vi "DataStorageSendDataEventRoutedMessage_Parse.vi"(8 "error in (no error)":errorcluster, 11 "Message":T10) -> (0 "error out":errorcluster, 1 "Body":T1, 2 "Header":T9, 3 "DataStorageSendDataEventRoutedMessage":T8)   [LabVIEW 2017]
uses:
  <vilib>/addons/InsightCM/MessageBus/Base/controls/Message.ctl
  <vilib>/addons/InsightCM/MessageBus/Base/controls/MessageHeader.ctl
  <vilib>/addons/InsightCM/MessageBus/Base/controls/KeyValuePair.ctl
  <vilib>/addons/InsightCM/MessageBus/MessageLibrary/DataStorage/controls/DataStorageSendDataEventRoutedMessage.ctl
  <vilib>/addons/InsightCM/MessageBus/MessageLibrary/DataStorage/controls/DataStorageSendDataEventRoutedMessageBody.ctl
  <vilib>/addons/InsightCM/MessageBus/Base/controls/DataEvent.ctl
  <vilib>/addons/InsightCM/MessageBus/Base/controls/DataSetMetadata.ctl
  <vilib>/addons/InsightCM/MessageBus/Base/controls/TrendPoint.ctl
  <vilib>/addons/InsightCM/MessageBus/Base/controls/TrendAlarmUpdate.ctl
  <vilib>/addons/InsightCM/MessageBus/Base/controls/TrendAlarmTransition.ctl
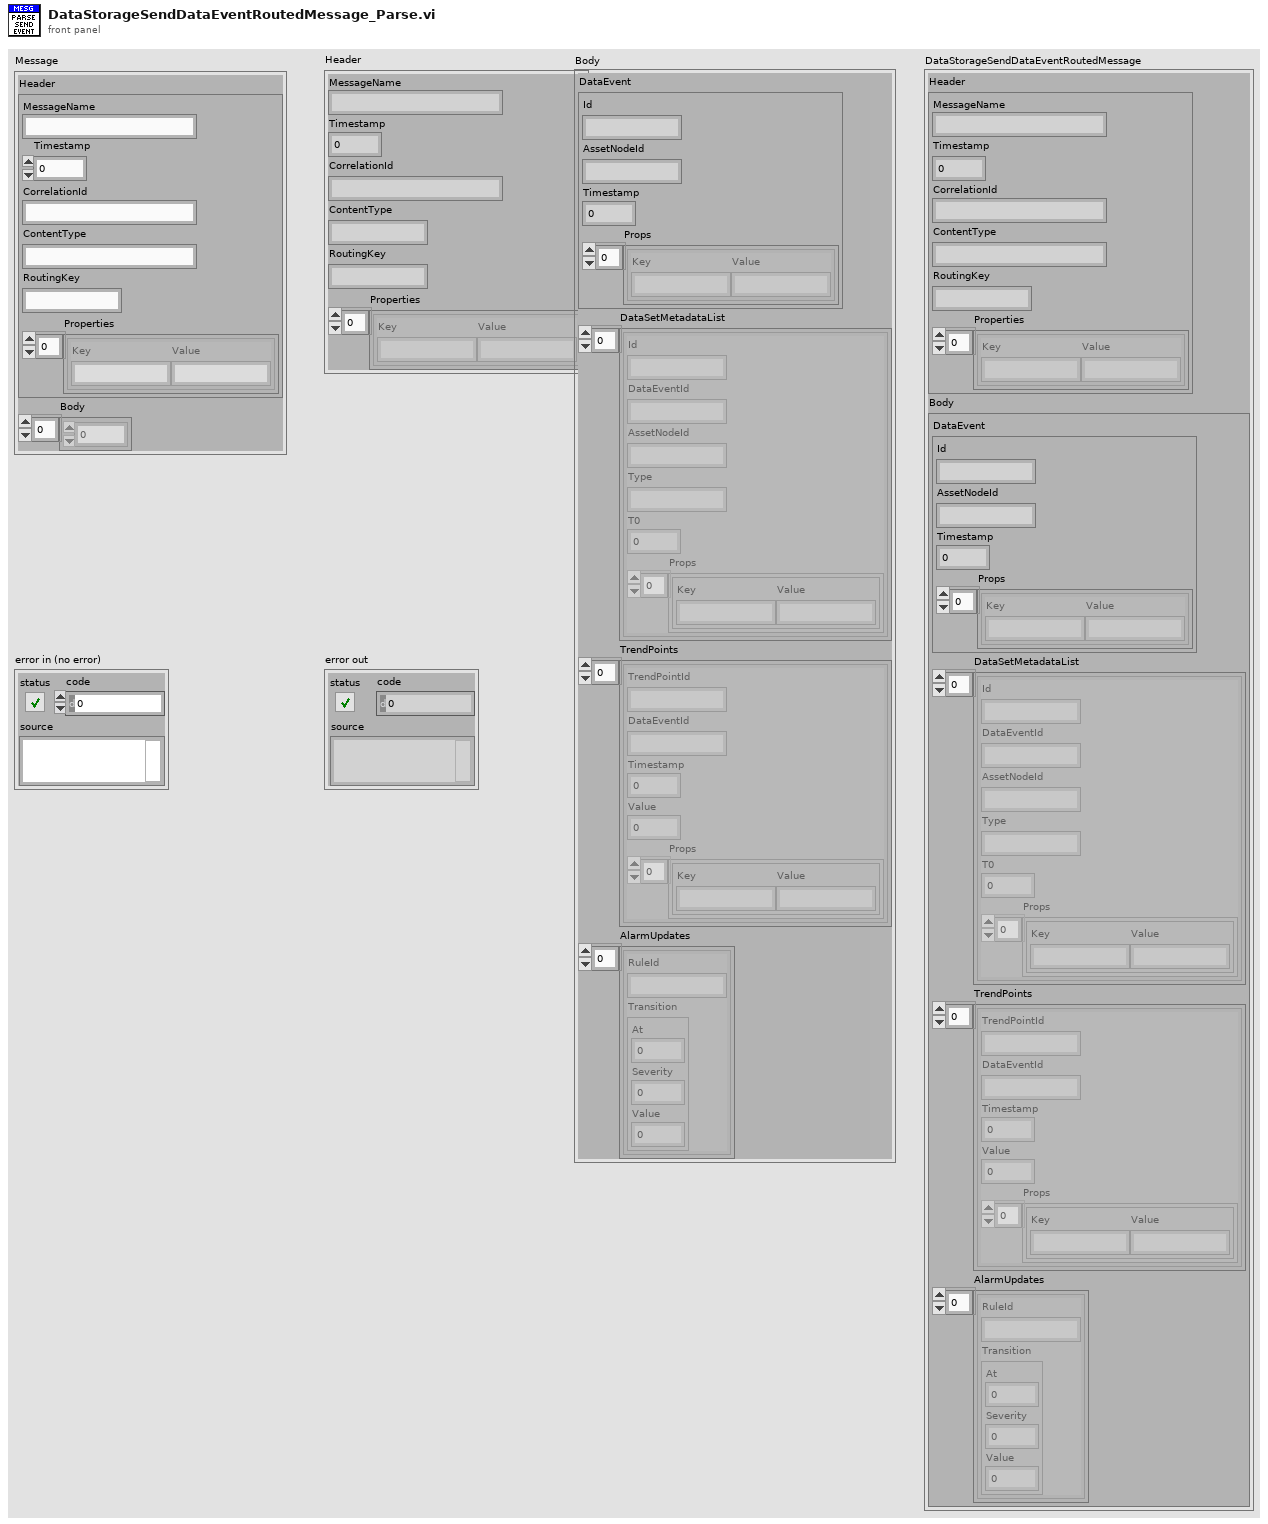
[diagram p1: front panel]
types:
  T1 = typedef "DataStorageSendDataEventRoutedMessageBody.ctl" = cluster{"DataEvent":T2, "DataSetMetadataList":T4[], "TrendPoints":T5[], "AlarmUpdates":T6[]}
  T2 = typedef "DataEvent.ctl" = cluster{"Id":string, "AssetNodeId":string, "Timestamp":i64, "Props":T3[]}
  T3 = typedef "KeyValuePair.ctl" = cluster{"Key":string, "Value":string}
  T4 = typedef "DataSetMetadata.ctl" = cluster{"Id":string, "DataEventId":string, "AssetNodeId":string, "Type":string, "T0":i64, "Props":T3[]}
  T5 = typedef "TrendPoint.ctl" = cluster{"TrendPointId":string, "DataEventId":string, "Timestamp":i64, "Value":dbl, "Props":T3[]}
  T6 = typedef "TrendAlarmUpdate.ctl" = cluster{"RuleId":string, "Transition":T7}
  T7 = typedef "TrendAlarmTransition.ctl" = cluster{"At":i64, "Severity":i32, "Value":dbl}
  T8 = typedef "DataStorageSendDataEventRoutedMessage.ctl" = cluster{"Header":T9, "Body":T1}
  T9 = typedef "MessageHeader.ctl" = cluster{"MessageName":string, "Timestamp":i64, "CorrelationId":string, "ContentType":string, "RoutingKey":string, "Properties":T3[]}
  T10 = typedef "Message.ctl" = cluster{"Header":T9, "Body":u8[]}
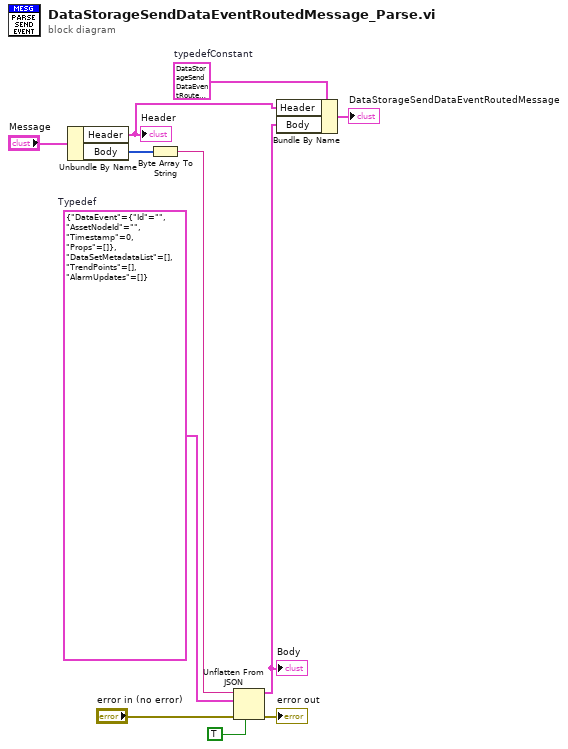
[diagram p0: block diagram]
diagram:
  w3 = T8 {"Header"={"MessageName"="", "Timestamp"=0, "CorrelationId"="", "ContentType"="", "RoutingKey"="", "Properties"=[]}, "Body"={"DataEvent"={"Id"="", "AssetNodeId"="", "Timestamp"=0, "Props"=[]}, "DataSetMetadataList"=[], "TrendPoints"=[], "AlarmUpdates"=[]}}  # typedefConstant
  w7 = T1 {"DataEvent"={"Id"="", "AssetNodeId"="", "Timestamp"=0, "Props"=[]}, "DataSetMetadataList"=[], "TrendPoints"=[], "AlarmUpdates"=[]}  # Typedef
  n1 = Unbundle By Name("Message") -> ("Header"=w9:T9, "Body"=w1:u8[])
  "Header" <- w9
  n2 = Byte Array To String(unsigned byte array=w1) -> (string=w6:string)
  n3 = Unflatten From JSON(JSON string=w6, type and defaults=w7, default null elements? (F)=TRUE, error in (no error)="error in (no error)") -> (value=w5:T1, error out=→"error out":errorcluster)  [unwired: 3 in]
  "Body" <- w5
  n4 = Bundle By Name(cluster=w3, "Header"=w9, "Body"=w5) -> (→"DataStorageSendDataEventRoutedMessage":T8)
